vi "Read Serial Data Chan_1.vi"(0 "FPGA Main IN":refnum<k20>, 11 "Error IN":errorcluster) -> (4 "FPGA VI OUT":refnum<k20>, 6 "#of Element Read":i32, 8 "String":string, 15 "Error OUT":errorcluster)   [LabVIEW 2011]
uses:
  <vilib>/Utility/error.llb/Error Cluster From Error Code.vi
  <vilib>/rvi/errors/niLvFpgaAdjustHostInterfaceError.vi
  <vilib>/RVI Host/nirviSupport.llb/nirviErrorClusterFromErrorCode.vi
  <vilib>/rvi/interface/nirviReadWriteControl/nirviReadWriteControl.xnode
  FPGA Bitfiles/JAGM_FPGATarget_FPGAMain_A31A659D.lvbitx
  FPGA Source/FPGA Main.vi
  <vilib>/rvi/interface/nirviMethod/nirviMethod.xnode
  <vilib>/rvi/interface/nirviMethod/StockFPGA_InlinedMethodWaitForSingleIRQ.vi
  <vilib>/FPGAPlugInAG/sbRIO-9606/niLvFpga_WaitOnIrq_sbRIO-9606.vi
  <vilib>/FPGAPlugInAG/sbRIO-9606/niLvFpga_AcknowledgeIrq_sbRIO-9606.vi
  NiFpgaLv.dll
  <vilib>/FPGAPlugInAG/sbRIO-9606/niLvFpga_ReadFifo_sbRIO-9606.vi
  <vilib>/rvi/errors/niLvFpgaMergeErrorWithErrorCode.vi
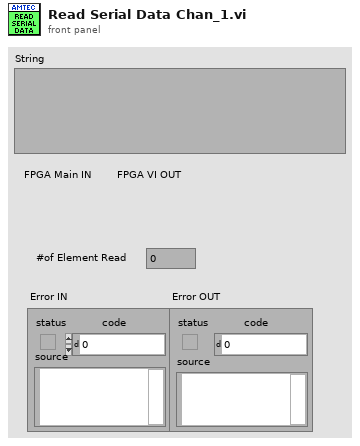
[diagram p1: front panel]
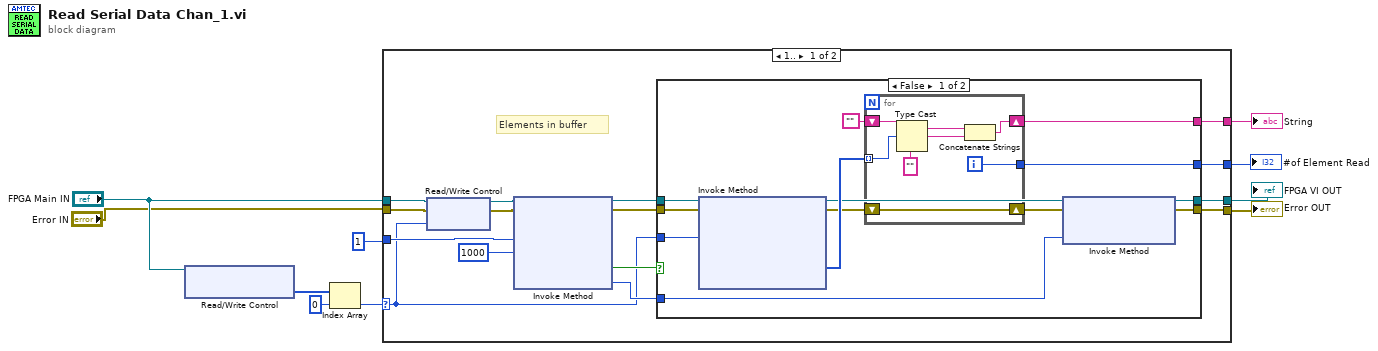
[diagram p0: block diagram]
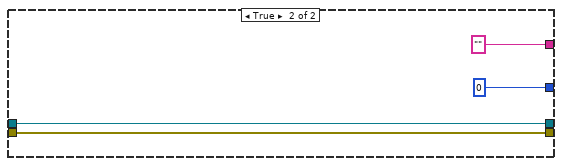
[diagram p2: hidden frame]
diagram:
  n1 = xnode "Read/Write Control"("FPGA VI Reference In"="FPGA Main IN") -> ("Element in Buffer"=w8:u32[])  [unwired: 1 in, 2 out]
  n2 = Index Array(array=w8, index=0) -> (element=w10:u32)
  n3 = case shown="1.." w10 {
    selector: w10 -> [w11 _]
    tunnel: "FPGA Main IN" -> [w15 w53]
    tunnel: "Error IN" -> [w14 w52]
    tunnel: [w23 w53] -> w1
    tunnel: [w24 w52] -> w4
    tunnel: [w25 ""] -> w3
    tunnel: 1 ("IRQ Number(s)") -> [w22 _]
    tunnel: [w18 0] -> w2
    frame 1.. {
      # "Elements in buffer"
      n4 = xnode "Read/Write Control"("FPGA VI Reference In"=w15, "error in"=w14, "Buffer#1"=w11) -> ("FPGA VI Reference Out"=w13:refnum<k20>, "error out"=w12:errorcluster)
      n5 = xnode ("Invoke Method")("FPGA VI Reference In"=w13, "error in"=w12, "IRQ Number(s)"=w22, "Timeout (ms)"=1000) -> ("FPGA VI Reference Out"=w20:refnum<k20>, "error out"=w19:errorcluster, "Timed Out"=w17:bool, "IRQ(s) Asserted"=w16:i32)
      n6 = case shown="False" w17 {
        tunnel: [w37 ""] -> w25
        tunnel: w11 -> [w36 _]
        tunnel: [w27 w48] -> w24
        tunnel: [w29 w49] -> w23
        tunnel: w20 -> [w35 w49]
        tunnel: w19 -> [w34 w48]
        tunnel: [w32 0] -> w18
        tunnel: w16 -> [w26 _]
        frame False {
          n7 = xnode ("Invoke Method")("FPGA VI Reference In"=w35, "error in"=w34, "Number of Elements"=w36) -> ("FPGA VI Reference Out"=w30:refnum<k20>, "error out"=w31:errorcluster, "Data"=w33:u8[])  [unwired: 1 in, 1 out]
          n8 = for {
            shift-right: [w45] -> w37
            shift-left: "" -> [w44]
            tunnel: w33 -> [w41] mode=indexing
            tunnel: [w40] -> w32
            shift-right: [w39] -> w28
            shift-left: w31 -> [w39]
            i -> [w40]
            n9 = Type Cast(type="", x=w41) -> (*(type *) &x=w42:string)
            n10 = Concatenate Strings(w44, w42) -> (w45:string)
          }
          n11 = xnode ("Invoke Method")("FPGA VI Reference In"=w30, "error in"=w28, "IRQ Number(s)"=w26) -> ("FPGA VI Reference Out"=w29:refnum<k20>, "error out"=w27:errorcluster)
        }
        frame True {
        }
      }
    }
    frame 0, Default {
      # "Buffer Empty"
    }
  }
  "Error OUT" <- w4
  "String" <- w3
  "FPGA VI OUT" <- w1
  "#of Element Read" <- w2
